vi "Pitch Change Detection.vi"(2 "Min Pitch":dbl, 3 "NavX refnum name":string="navX") -> ()   [LabVIEW 2015]
uses:
  Pitch Change Typedef.ctl
  navX Library v2/navX Library v2.lvlib
panel:
  in  "stop":bool
  in  "Pitch":dbl
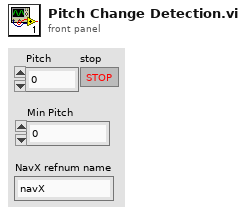
[diagram p1: front panel]
types:
  T1 = typedef "Pitch Change Typedef.ctl" = enum16{"Flat", "Going up Forwards", "Going up Backwards", "Going down", "Crossed Sucessfully"}
  T2 = typedef "navX Library v2.lvlib/Z900_navX_DeviceTypeDef.ctl" = cluster{"Interface":cluster{"Protocol":T3, "Update Rate (4Hz-60Hz)":u8, "navX Open TypeDef":variant}, "Notify Packet":refnum<notifier>, "Loop VI Refnum":refnum<vi>, "Ready to Close Occurrence Refnum":refnum<k4>}
  T3 = typedef "navX Library v2.lvlib/Z900_navX_ProtocolTypeDef.ctl" = enum16{"SERIAL", "I2C", "SPI"}
  T4 = cluster{"Yaw":dbl, "Roll":dbl, "Pitch":dbl, "Heading":dbl, "Fused Heading":dbl}
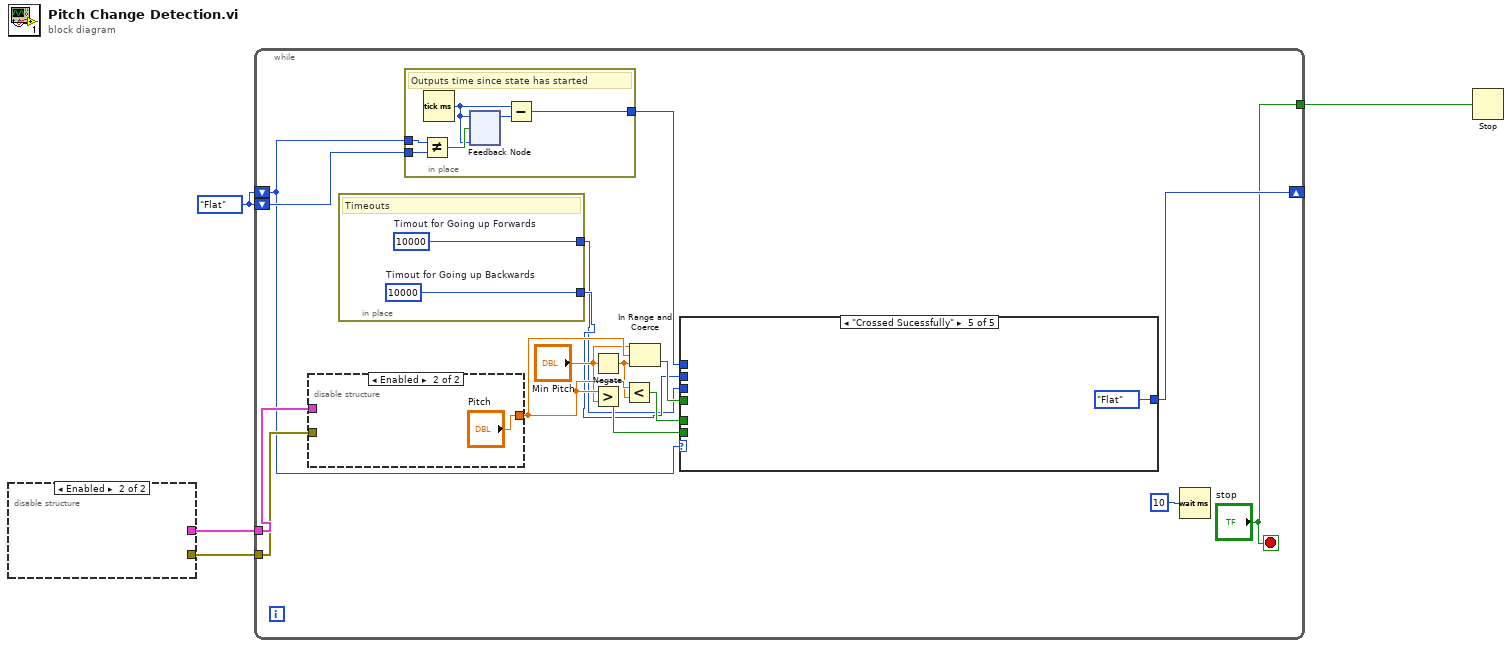
[diagram p0: block diagram]
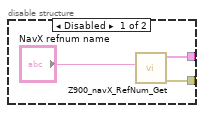
[diagram p2: hidden frame]
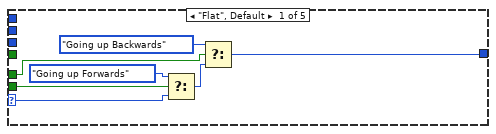
[diagram p3: hidden frame]
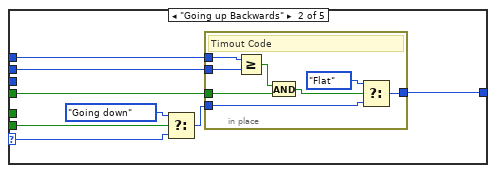
[diagram p4: hidden frame]
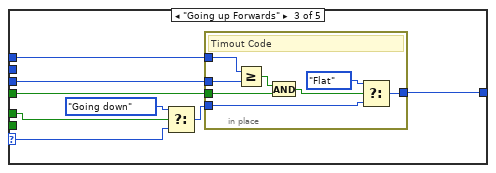
[diagram p5: hidden frame]
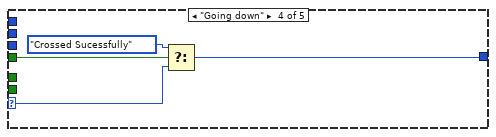
[diagram p6: hidden frame]
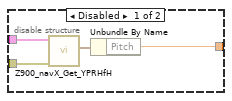
[diagram p7: hidden frame]
diagram:
  w2 = Pitch_Change_Typedef."Flat"
  n1 = disable-structure shown="Enabled" {
    disable-tunnel: [w6 _] -> w4
    disable-tunnel: [w5 _] -> w3
    frame Disabled {
      n2 = call "Z900_navX_RefNum_Get.vi"("refnum name"="NavX refnum name") -> ("error out"=w5:errorcluster, "navX Device"=w6:T2)  [unwired: 9 in]
    }
    frame Enabled {
    }
  }
  n3 = while {
    shift-right: [w13] -> _
    shift-left: w2 -> [w14]
    tunnel: w4 -> [w17]
    tunnel: w3 -> [w16]
    shift-left: w2 -> [w15]
    tunnel: ["stop"] -> w1
    stop <- "stop" stop-if-true
    n4 = disable-structure shown="Enabled" {
      disable-tunnel: [w78 "Pitch"] -> w23
      disable-tunnel: w17 -> [w77 _]
      disable-tunnel: w16 -> [w76 _]
      frame Disabled {
        n5 = call "Z900_navX_Get_YPRHfH.vi"("error in (no error)"=w76, "navX Device"=w77) -> ("YRPHfH"=w79:T4)  [unwired: 6 in, 3 out]
        n6 = Unbundle By Name(w79) -> ("Pitch"=w78:dbl)
      }
      frame Enabled {
      }
    }
    n7 = in-place {
      in-place-border: [w25] -> w9
      in-place-border: [w24] -> w8
      w24 = u32 10000  # Timout for Going up Forwards
      w25 = u32 10000  # Timout for Going up Backwards
      # "Timeouts"
    }
    n8 = in-place {
      in-place-border: w15 -> [w31]
      in-place-border: w14 -> [w30]
      in-place-border: [w27] -> w10
      # "Outputs time since state has started"
      n9 = Not Equal?(x=w30, y=w31) -> (x != y?=w29:bool)
      n10 = Tick Count (ms)() -> (millisecond timer value=w26:u32)
      n11 = feedback #1(w26) -> (w28:u32)
      n12 = feedback-in #1(w26, w29) -> ()
      n13 = Subtract(x=w26, y=w28) -> (x-y=w27:u32)
    }
    n14 = Negate(x="Min Pitch") -> (-x=w11:dbl)
    n15 = Greater?(x=w23, y="Min Pitch") -> (0:w20:bool)
    n16 = Less?(x=w23, y=w11) -> (x < y?=w19:bool)
    n17 = In Range and Coerce(upper limit="Min Pitch", x=w23, lower limit=w11) -> (In Range?=w18:bool)  [unwired: 1 out]
    n18 = case shown="\"Crossed Sucessfully\"" w14 {
      selector: w14 -> [w37 w46 w62 w74 _]
      tunnel: w20 -> [w38 w45 _ _ _]
      tunnel: w19 -> [w35 _ w60 _ _]
      tunnel: [w32 w42 w57 w72 Pitch_Change_Typedef."Flat"] -> w13
      tunnel: w18 -> [_ w44 w58 w71 _]
      tunnel: w10 -> [_ w40 w59 _ _]
      tunnel: w9 -> [_ w41 _ _ _]
      tunnel: w8 -> [_ _ w55 _ _]
      frame "Flat", Default {
        n19 = Select(t=Pitch_Change_Typedef."Going up Forwards", s=w38, f=w37) -> (s? t:f=w36:T1)
        n20 = Select(t=Pitch_Change_Typedef."Going up Backwards", s=w35, f=w36) -> (s? t:f=w32:T1)
      }
      frame "Going up Backwards" {
        n21 = Select(t=Pitch_Change_Typedef."Going down", s=w45, f=w46) -> (s? t:f=w43:T1)
        n22 = in-place {
          in-place-border: w44 -> [w54]
          in-place-border: w43 -> [w50]
          in-place-border: [w49] -> w42
          in-place-border: w41 -> [w48]
          in-place-border: w40 -> [w47]
          # "Timout Code"
          n23 = Greater Or Equal?(x=w47, y=w48) -> (x >= y?=w53:bool)
          n24 = And(x=w53, y=w54) -> (x .and. y?=w52:bool)
          n25 = Select(t=Pitch_Change_Typedef."Flat", s=w52, f=w50) -> (s? t:f=w49:T1)
        }
      }
      frame "Going up Forwards" {
        n26 = Select(t=Pitch_Change_Typedef."Going down", s=w60, f=w62) -> (s? t:f=w56:T1)
        n27 = in-place {
          in-place-border: w58 -> [w70]
          in-place-border: w56 -> [w66]
          in-place-border: [w65] -> w57
          in-place-border: w55 -> [w64]
          in-place-border: w59 -> [w63]
          # "Timout Code"
          n28 = Greater Or Equal?(x=w63, y=w64) -> (x >= y?=w69:bool)
          n29 = And(x=w69, y=w70) -> (x .and. y?=w68:bool)
          n30 = Select(t=Pitch_Change_Typedef."Flat", s=w68, f=w66) -> (s? t:f=w65:T1)
        }
      }
      frame "Going down" {
        n31 = Select(t=Pitch_Change_Typedef."Crossed Sucessfully", s=w71, f=w74) -> (s? t:f=w72:T1)
      }
      frame "Crossed Sucessfully" {
      }
    }
    n32 = Wait (ms)(milliseconds to wait=u32 10) -> ()  [unwired: 1 out]
  }
  n33 = Stop(stop? (T)=w1) -> ()
